vi "reward_behavior_no_TO.vi"() -> ()   [LabVIEW 2019]
doc: "The myRIO Project template acquires acceleration data from the onboard accelerometer and displays the changes of acceleration values in a waveform chart."
uses:
  <vilib>/Analysis/Matrix/Datatypes/RealMatrix.ctl
  <vilib>/myRIO/Common/Instrument Driver Framework/myRIO v1.0/Encoder/typedefs/Encoder Signal Mode.ctl
  <vilib>/myRIO/Instrument Drivers/Onboard IO/Encoder/typedefs/Encoder Reference.ctl
  <vilib>/myRIO/Common/Instrument Driver Framework/Utilities/typedefs/myRIO Generic Hardware Reference.ctl
  <vilib>/myRIO/Common/Instrument Driver Framework/Utilities/typedefs/Hardware Version Enum.ctl
  <vilib>/myRIO/Common/Instrument Driver Framework/Utilities/typedefs/myRIO v1.0 Reference.ctl
  <vilib>/myRIO/Common/Instrument Driver Framework/Utilities/typedefs/Generic FPGA Reference.ctl
  <vilib>/myRIO/Common/Instrument Driver Framework/myRIO v1.0/Encoder/typedefs/Encoder Channels Enum.ctl
  <vilib>/myRIO/Common/Instrument Driver Framework/myRIO v1.0/Encoder/typedefs/Encoder Configuration v1.0.ctl
  <vilib>/userdefined/High Color/nirio_resource_hc.ctl
  <vilib>/myRIO/Instrument Drivers/Onboard IO/DIO/typedefs/DIO Reference.ctl
  <vilib>/myRIO/Common/Instrument Driver Framework/myRIO v1.0/DIO/typedefs/DIO Channels List.ctl
  <vilib>/myRIO/Common/Instrument Driver Framework/myRIO v1.0/DIO/typedefs/DIO Channels Enum.ctl
  <vilib>/myRIO/Common/Instrument Driver Framework/Utilities/vis/Is FPGA Ref Available.vi
  <vilib>/myRIO/Common/Instrument Driver Framework/myRIO v1.0/Encoder/vis/myRIO v1.1 Open Encoder.vi
  <vilib>/myRIO/Instrument Drivers/Onboard IO/Encoder/vis/Read.vi
  <vilib>/myRIO/Common/Instrument Driver Framework/myRIO v1.0/DIO/vis/myRIO v1.1 Open DIO.vi
  <vilib>/myRIO/Instrument Drivers/Onboard IO/DIO/vis/Write.vi
  <vilib>/myRIO/Instrument Drivers/Onboard IO/DIO/vis/Read.vi
  <vilib>/myRIO/Common/Instrument Driver Framework/Utilities/vis/Validate Channels.vi
  <vilib>/myRIO/Common/Instrument Driver Framework/myRIO v1.0/Encoder/vis/myRIO v1.0 Reserve Encoder.vi
  <vilib>/myRIO/Common/Instrument Driver Framework/myRIO v1.0/DIO/vis/myRIO v1.0 Reserve DIO.vi
  <vilib>/myRIO/Common/Instrument Driver Framework/myRIO v1.0/Encoder/vis/myRIO v1.0 Build MUX Configuration Encoder.vi
  <vilib>/myRIO/Common/Instrument Driver Framework/myRIO v1.0/Resource Manager/vis/myRIO v1.0 Reserve Channel List.vi
  <vilib>/myRIO/Common/Instrument Driver Framework/myRIO v1.0/DIO/vis/myRIO v1.0 Build MUX Configuration DIO.vi
  <vilib>/myRIO/Common/Instrument Driver Framework/myRIO v1.0/Resource Manager/vis/myRIO v1.0 Create Configuration List.vi
  <vilib>/myRIO/Common/Instrument Driver Framework/myRIO v1.0/Resource Manager/vis/myRIO v1.0 Reserve Channel.vi
  <vilib>/myRIO/Common/Instrument Driver Framework/myRIO v1.0/Resource Manager/vis/myRIO v1.0 Unreserve Channel.vi
  <vilib>/myRIO/Common/Instrument Driver Framework/myRIO v1.0/Resource Manager/vis/myRIO v1.0 Build Mutex Name.vi
  <vilib>/Utility/VariantDataType/GetNumericInfo.vi
  <vilib>/Utility/error.llb/Error Cluster From Error Code.vi
  <vilib>/myRIO/Common/Instrument Driver Framework/myRIO v1.0/myRIO v1.1 Open.vi
  <vilib>/myRIO/Common/Instrument Driver Framework/Utilities/vis/IO Manager.vi
  <vilib>/myRIO/Common/Instrument Driver Framework/Utilities/vis/Configuration Manager.vi
  <vilib>/myRIO/Common/Instrument Driver Framework/myRIO v1.0/Resource Manager/vis/myRIO v1.0 Configure IO.vi
  <vilib>/myRIO/Common/Instrument Driver Framework/myRIO v1.0/myRIO v1.0 Close.vi
  <vilib>/myRIO/Common/Instrument Driver Framework/myRIO v1.0/Encoder/vis/myRIO v1.0 Configure Encoder.vi
  <vilib>/myRIO/Common/Instrument Driver Framework/myRIO v1.0/Encoder/vis/myRIO v1.0 Read Encoder.vi
  <vilib>/myRIO/Common/Instrument Driver Framework/myRIO v1.0/DIO/vis/myRIO v1.0 Read DIO.vi
  <vilib>/myRIO/Common/Instrument Driver Framework/myRIO v1.0/DIO/vis/myRIO v1.0 Write DIO.vi
  <vilib>/myRIO/Express VI/Onboard IO/Encoder/Encoder Express VI.xnode
  <vilib>/myRIO/Instrument Drivers/Onboard IO/Encoder/vis/myRIO Encoder Open.xnode
  <vilib>/myRIO/Express VI/Onboard IO/DI/DI Express VI.xnode
  <vilib>/myRIO/Instrument Drivers/Onboard IO/DIO/vis/myRIO DIO Open.xnode
  <vilib>/myRIO/Express VI/Onboard IO/DO/DO Express VI.xnode
  <vilib>/myRIO/Instrument Drivers/Onboard IO/Encoder/Encoder.lvlib
  <vilib>/myRIO/Instrument Drivers/Onboard IO/DIO/DIO.lvlib
  <vilib>/Analysis/Matrix/NI_Matrix.lvlib
panel:
  out "Timings":dbl[](array[numeric])
  out "ISI":dbl
  out "ISI start time":dbl
  out "Time_out":bool=TRUE
  out "Time since lick":dbl
  out "Time of last lick":dbl
  out "Rewarded trials":dbl[](array[numeric])
  out "Rewards":u16
  out "Active Trial":bool
  out "Array temp2":T1
  out "Stimuli Loaded":bool
  out "Stim_ID":dbl[](array[numeric])
  out "Reward_mat":dbl[](array[numeric])
  out "Reward":bool=TRUE
  out "Frame clock":i32
  out "Licks":u32
  out "Lick":bool
  out "Time":dbl
  out "Stop":bool
  in  "Frames to collect":u32
  out "Overflow?":bool
  out "Counter Value":i32
  out "Velocity":dbl
  out "Velocity Plot":dbl[](graph)
  out "Velocity array":dbl[](array[numeric])
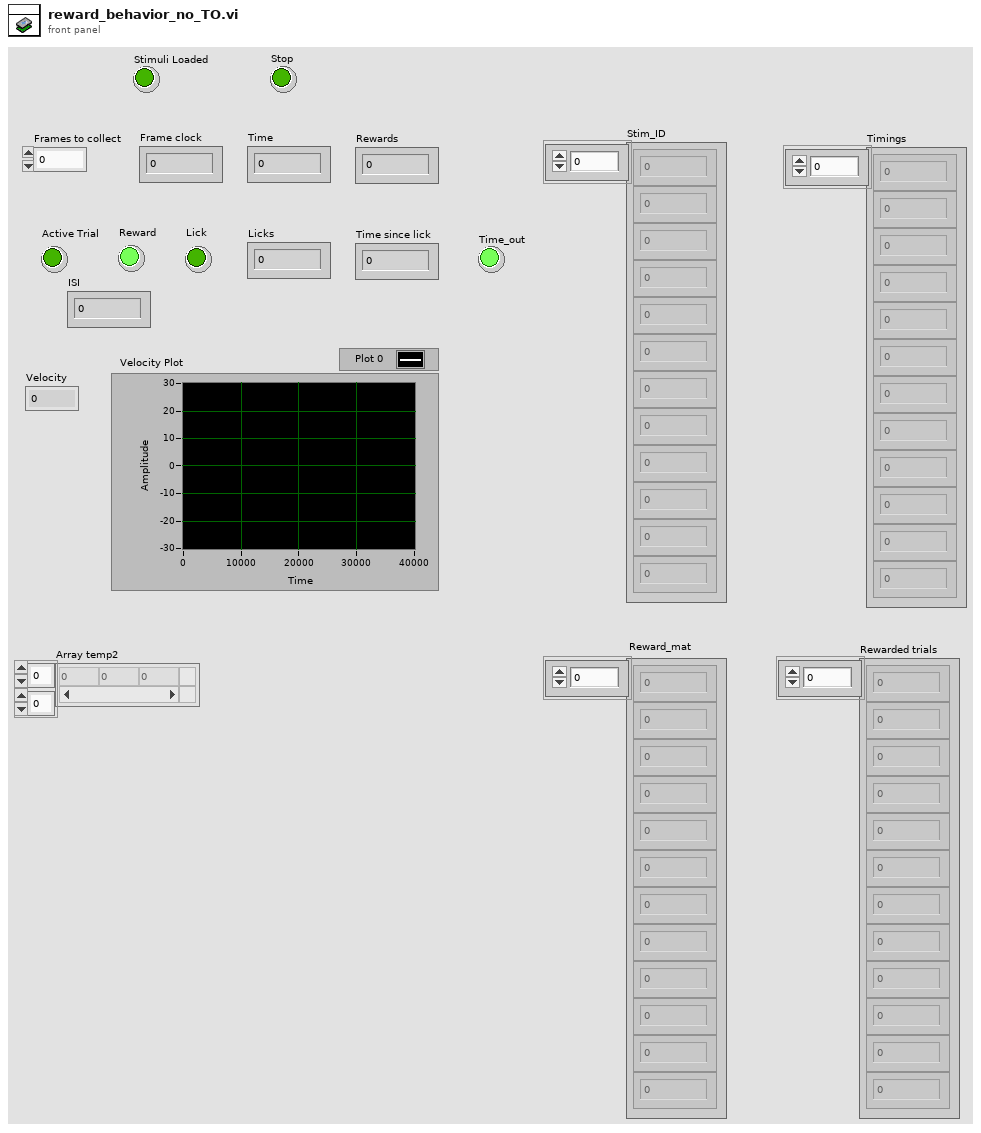
[diagram p1: front panel]
types:
  T1 = typedef "NI_Matrix.lvlib/RealMatrix.ctl" = dbl[][]
  T2 = typedef "Encoder.lvlib/Encoder Reference.ctl" = cluster{"myRIO Reference":T3, "Encoder Channels Enum":T7}
  T3 = typedef "myRIO Generic Hardware Reference.ctl" = cluster{"myRIO Model":T4, "myRIO Hardware Reference":T5}
  T4 = typedef "Hardware Version Enum.ctl" = enum16{"Unknown", "myRIO-1900", "myRIO-1950", "roboRIO", "NI ELVIS RIO CM", "ELVIS III"}
  T5 = typedef "myRIO v1.0 Reference.ctl" = cluster{"Generic FPGA Reference":T6, "Allow multiple opens":bool}
  T6 = typedef "Generic FPGA Reference.ctl" = refnum<k20>
  T7 = typedef "Encoder Channels Enum.ctl" = enum16{"Not Connected", "C/ENC0", "C/ENC1", "A/ENC", "A/ENC0", "A/ENC1", "A/ENC2", "A/ENC3", "A/ENC4", "A/ENC5", "A/ENC6", "A/ENC7", "A/ENC8", "A/ENC9", "B/ENC", "B/ENC0", "B/ENC1", "B/ENC2", "B/ENC3", "B/ENC4", "B/ENC5", "B/ENC6", "B/ENC7", "B/ENC8", "B/ENC9", "DIO/ENC0", "DIO/ENC1", "DIO/ENC2", "DIO/ENC3", "DIO/ENC4"}
  T8 = typedef "Encoder Signal Mode.ctl" = enum16{"Quadrature phase signal", "Step and direction signal"}
  T9 = typedef "nirio_resource_hc.ctl" = tag
  T10 = typedef "DIO.lvlib/DIO Reference.ctl" = cluster{"myRIO Reference":T3, "DIO Channels List":T11}
  T11 = typedef "DIO Channels List.ctl" = T12[]
  T12 = typedef "DIO Channels Enum.ctl" = enum16{"Not Connected", "C/DIO0", "C/DIO1", "C/DIO2", "C/DIO3", "C/DIO4", "C/DIO5", "C/DIO6", "C/DIO7", "A/DIO0", "A/DIO1", "A/DIO2", "A/DIO3", "A/DIO4", "A/DIO5", "A/DIO6", "A/DIO7", "A/DIO8", "A/DIO9", "A/DIO10", "A/DIO11", "A/DIO12", "A/DIO13", "A/DIO14", "A/DIO15", "A/DIO16", "A/DIO17", "A/DIO18", "A/DIO19", "B/DIO0", "B/DIO1", "B/DIO2", "B/DIO3", "B/DIO4", "B/DIO5", "B/DIO6", "B/DIO7", "B/DIO8", "B/DIO9", "B/DIO10", "B/DIO11", "B/DIO12", "B/DIO13", "B/DIO14", "B/DIO15", "B/DIO16", "B/DIO17", "B/DIO18", "B/DIO19", "LED0", "LED1", "LED2", "LED3", "Button0", "DIO/DIO0", "DIO/DIO1", "DIO/DIO2", "DIO/DIO3", "DIO/DIO4", "DIO/DIO5", "DIO/DIO6", "DIO/DIO7", "DIO/DIO8", "DIO/DIO9", "SPI/CS0", "SPI/CS1", "SPI/CS2", "SPI/CS3", "LED RADIO (Green)", "LED RADIO (Red)", "LED COMM (Green)", "LED COMM (Red)", "LED MODE (Green)", "LED MODE (Red)"}
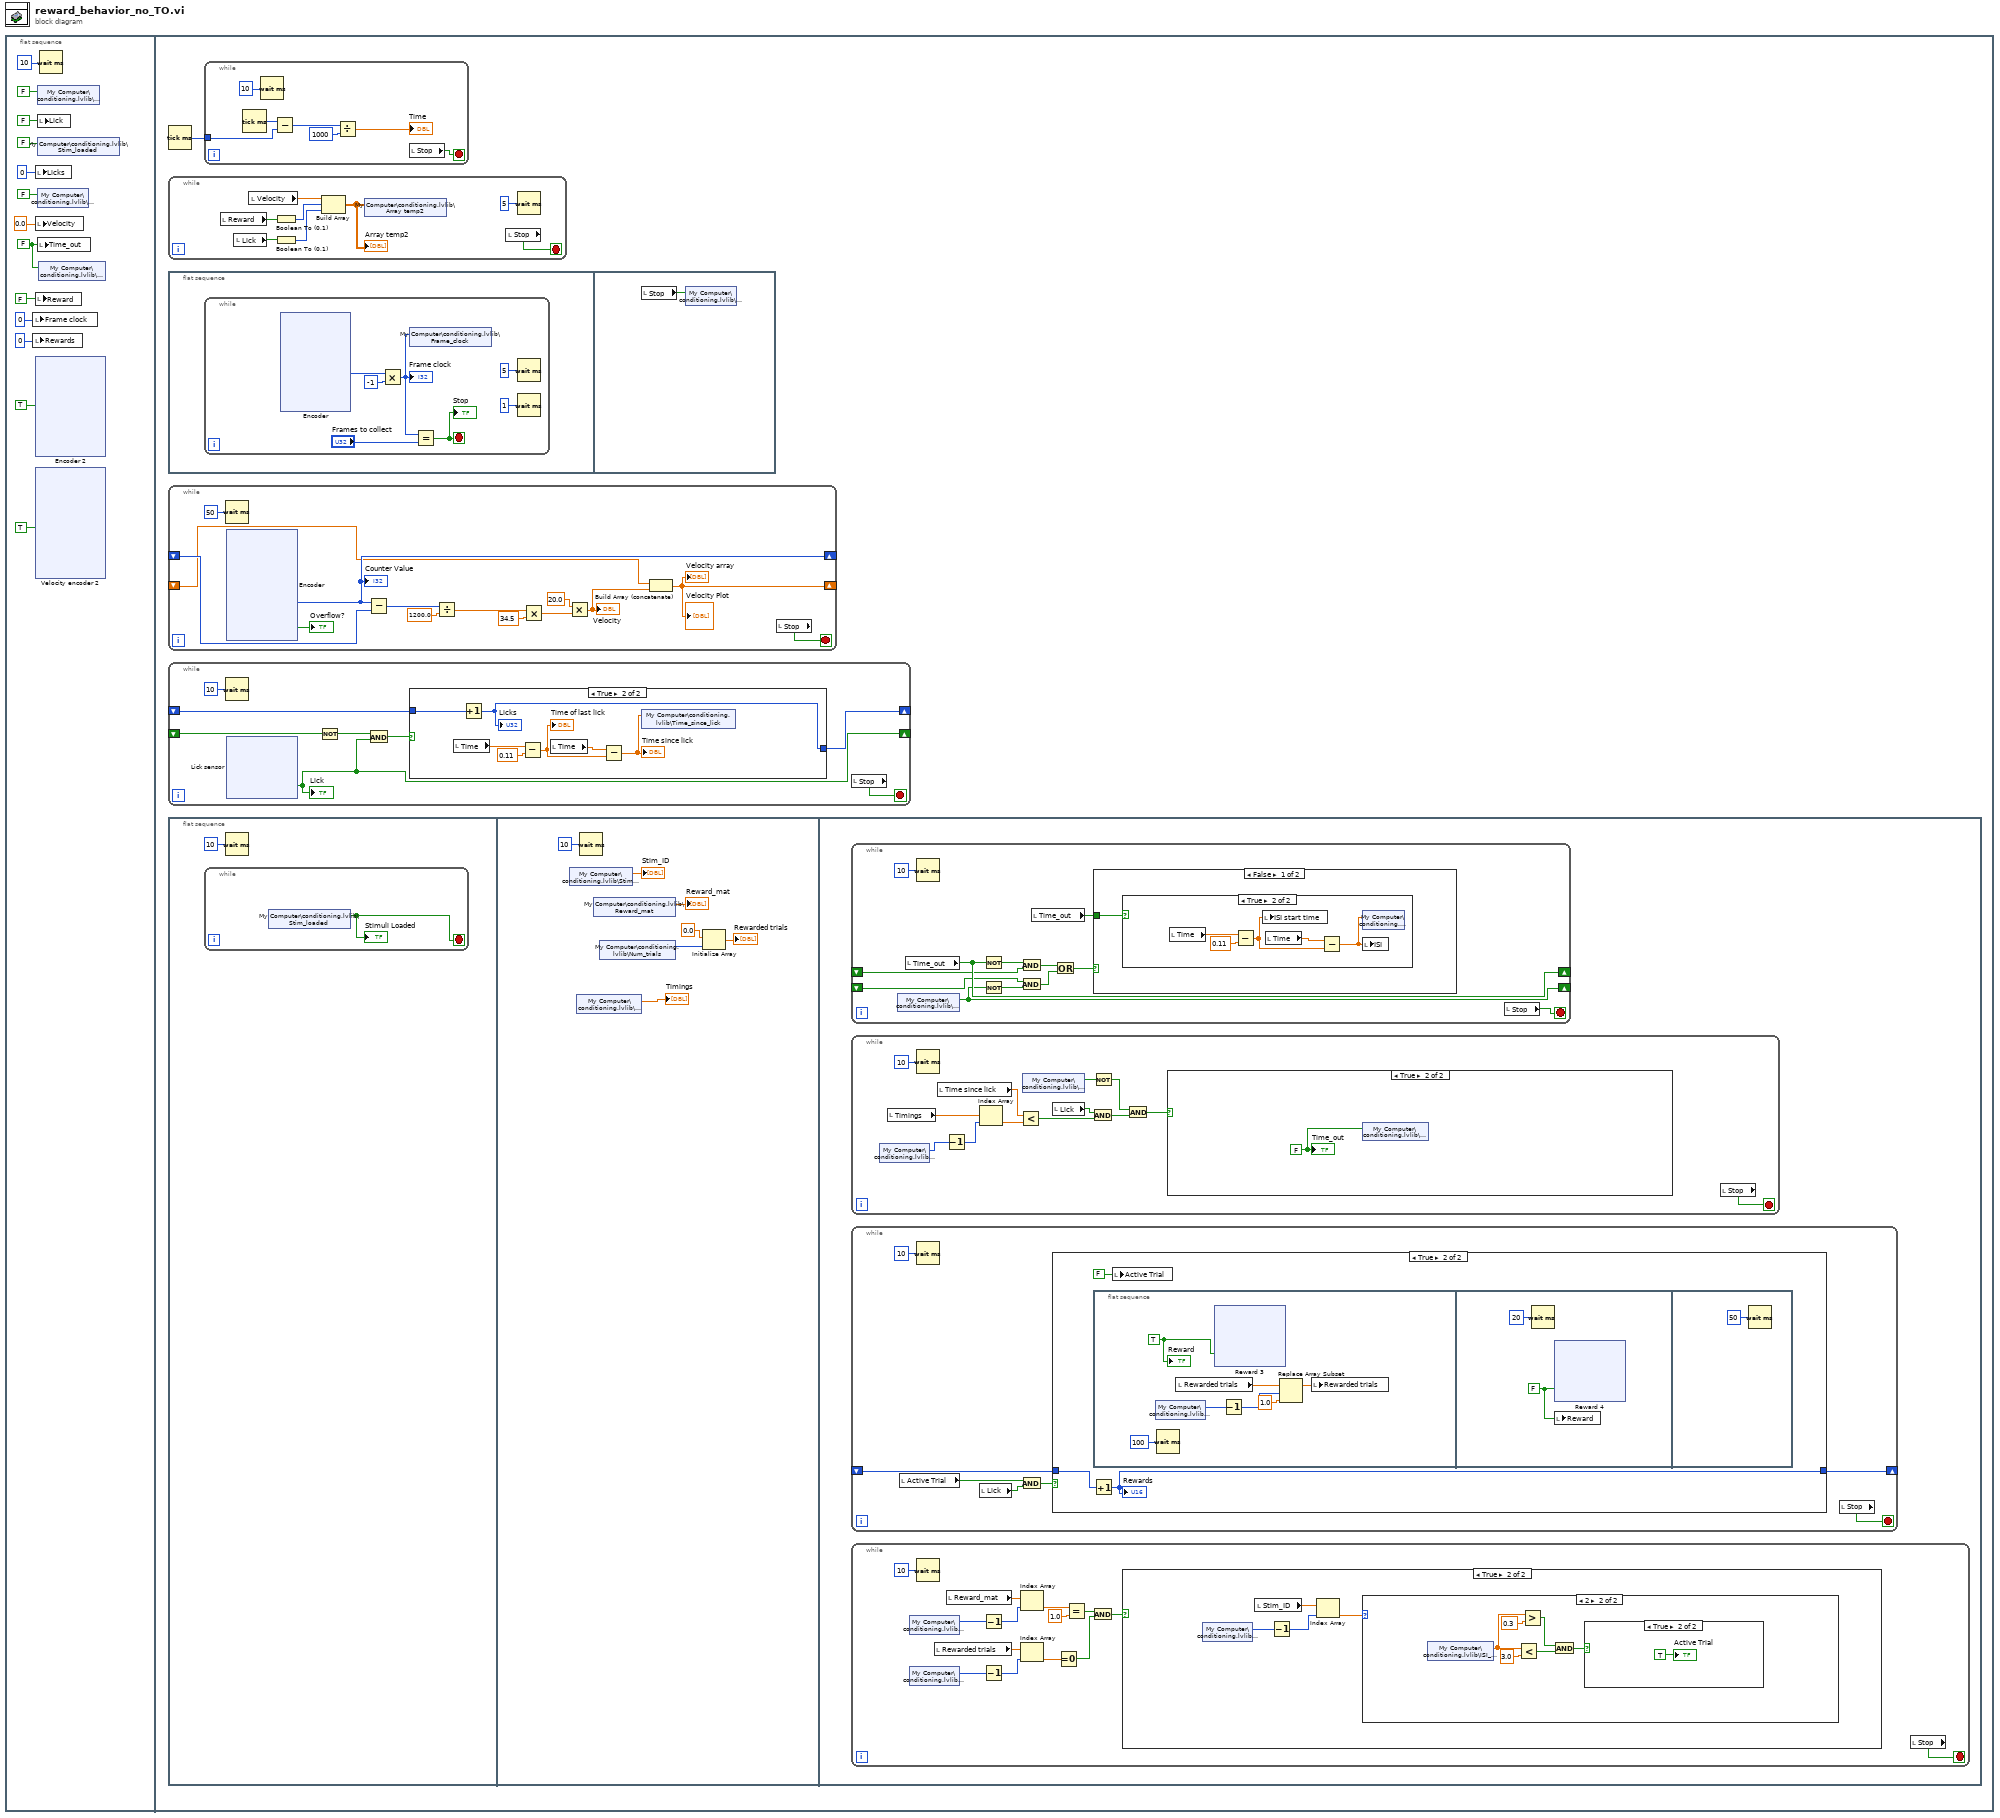
[diagram p0: block diagram]
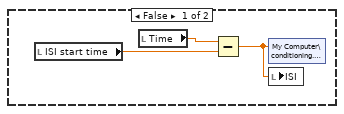
[diagram p3: hidden frame]
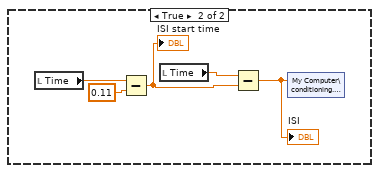
[diagram p4: hidden frame]
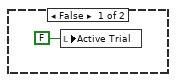
[diagram p5: hidden frame]
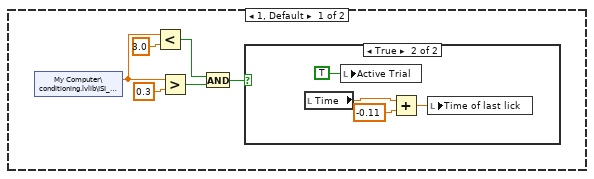
[diagram p6: hidden frame]
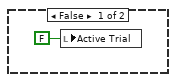
[diagram p7: hidden frame]
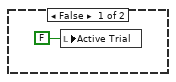
[diagram p8: hidden frame]
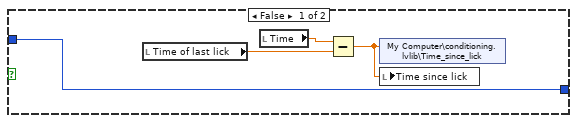
[diagram p10: hidden frame]
diagram:
  n1 = flat-sequence {
    frame #0 {
      w1 = FALSE ("Time_out")
      n2 = local write "Frame clock"(u32 0 ("Frames")) -> ()
      n3 = local write "Rewards"(u16 0 ("Rewards")) -> ()
      n4 = local write "Licks"(u32 0 ("Licks")) -> ()
      n5 = local write "Velocity"(0.0 ("Velocity")) -> ()
      n6 = local write "Reward"(FALSE ("Give reward")) -> ()
      n7 = xnode "Encoder 2"("Reset Counter"=TRUE) -> ()  [unwired: 1 in, 4 out]
      n8 = xnode "Velocity encoder 2"("Reset Counter"=TRUE) -> ()  [unwired: 1 in, 4 out]
      n9 = shared-variable "My Computer\\conditioning.lvlib\\Display"(FALSE ("Display")) -> ()  [unwired: 1 in, 1 out]
      n10 = local write "Lick"(FALSE ("Lick")) -> ()
      n11 = shared-variable "My Computer\\conditioning.lvlib\\Stim_loaded"(FALSE ("Stim_loaded")) -> ()  [unwired: 1 in, 1 out]
      n12 = shared-variable "My Computer\\conditioning.lvlib\\Stop"(FALSE ("Stop")) -> ()  [unwired: 1 in, 1 out]
      n13 = local write "Time_out"(w1) -> ()
      n14 = shared-variable "My Computer\\conditioning.lvlib\\Timeout"(w1) -> ()  [unwired: 1 in, 1 out]
      n15 = Wait (ms)(milliseconds to wait=u32 10) -> ()  [unwired: 1 out]
    }
    frame #1 {
      n16 = Tick Count (ms)() -> (millisecond timer value=w106:u32)
      n17 = while {
        stop <- w108 stop-if-true
        n18 = local read "Reward"() -> (w113:bool)
        n19 = local read "Lick"() -> (w114:bool)
        n20 = local read "Velocity"() -> (w112:dbl)
        n21 = Boolean To (0,1)(Boolean=w113) -> (0, 1=w111:i16)
        n22 = Boolean To (0,1)(Boolean=w114) -> (0, 1=w110:i16)
        n23 = Build Array(w112, w111, w110) -> (w107:T1)
        "Array temp2" <- w107
        n24 = shared-variable "My Computer\\conditioning.lvlib\\Array temp2"(w107) -> ()  [unwired: 1 in, 1 out]
        n25 = local read "Stop"() -> (w108:bool)
        n26 = Wait (ms)(milliseconds to wait=u32 5) -> ()  [unwired: 1 out]
      }
      n27 = flat-sequence {
        frame #0 {
          n28 = while {
            stop <- w294 stop-if-true
            n29 = xnode "Encoder"() -> ("Counter Value"=w298:i32)  [unwired: 2 in, 3 out]
            n30 = Multiply(x=w298, y=-1) -> (x*y=w293:i32)
            "Frame clock" <- w293
            n31 = shared-variable "My Computer\\conditioning.lvlib\\Frame_clock"(w293) -> ()  [unwired: 1 in, 1 out]
            n32 = Equal?(x=w293, y="Frames to collect") -> (x = y?=w294:bool)
            "Stop" <- w294
            n33 = Wait (ms)(milliseconds to wait=u32 5) -> ()  [unwired: 1 out]
            n34 = Wait (ms)(milliseconds to wait=u32 1) -> ()  [unwired: 1 out]
          }
        }
        frame #1 {
          n35 = local read "Stop"() -> (w346:bool)
          n36 = shared-variable "My Computer\\conditioning.lvlib\\Stop"(w346) -> ()  [unwired: 1 in, 1 out]
        }
      }
      n37 = while {
        shift-right: [w411] -> _
        shift-left: _ -> [w412]
        shift-right: [w403] -> _
        shift-left: _ -> [w402]
        stop <- w401 stop-if-true
        n38 = Wait (ms)(milliseconds to wait=u32 50) -> ()  [unwired: 1 out]
        n39 = xnode "Encoder"() -> ("Counter Value"=w411:i32, "Overflow?"=→"Overflow?":bool)  [unwired: 2 in, 2 out]
        "Counter Value" <- w411
        n40 = Subtract(x=w411, y=w412) -> (x-y=w404:i32)
        n41 = Divide(x=w404, y=1200.0 ("600")) -> (x/y=w409:dbl)
        n42 = Multiply(x=w409, y=34.5) -> (x*y=w407:dbl)
        n43 = Multiply(x=20.0, y=w407) -> (x*y=w405:dbl)
        "Velocity" <- w405
        n44 = Build Array (concatenate)(w402, w405) -> (w403:dbl[])
        "Velocity Plot" <- w403
        "Velocity array" <- w403
        n45 = local read "Stop"() -> (w401:bool)
      }
      n46 = while {
        shift-right: [w353] -> _
        shift-left: _ -> [w352]
        shift-right: [w347] -> _
        shift-left: _ -> [w350]
        stop <- w351 stop-if-true
        n47 = Wait (ms)(milliseconds to wait=u32 10) -> ()  [unwired: 1 out]
        n48 = xnode "Lick sensor"() -> ("C/DIO1 (DIO1)"=w347:bool)  [unwired: 1 in, 1 out]
        "Lick" <- w347
        n49 = Not(x=w350) -> (.not. x?=w349:bool)
        n50 = And(x=w349, y=w347) -> (x .and. y?=w348:bool)
        n51 = case shown="True" w348 {
          tunnel: [w358 w365] -> w353
          tunnel: w352 -> [w358 w364]
          frame False {
            n52 = local read "Time of last lick"() -> (w356:dbl)
            n53 = local read "Time"() -> (w357:dbl)
            n54 = Subtract(x=w357, y=w356) -> (x-y=w355:dbl)
            n55 = shared-variable "My Computer\\conditioning.lvlib\\Time_since_lick"(w355) -> ()  [unwired: 1 in, 1 out]
            n56 = local write "Time since lick"(w355) -> ()
          }
          frame True {
            n57 = local read "Time"() -> (w361:dbl)
            n58 = Increment(x=w364) -> (x+1=w365:u32)
            "Licks" <- w365
            n59 = Subtract(x=w361, y=0.11) -> (x-y=w359:dbl)
            "Time of last lick" <- w359
            n60 = local read "Time"() -> (w363:dbl)
            n61 = Subtract(x=w363, y=w359) -> (x-y=w362:dbl)
            "Time since lick" <- w362
            n62 = shared-variable "My Computer\\conditioning.lvlib\\Time_since_lick"(w362) -> ()  [unwired: 1 in, 1 out]
          }
        }
        n63 = local read "Stop"() -> (w351:bool)
      }
      n64 = flat-sequence {
        frame #0 {
          n65 = while {
            stop <- w116 stop-if-true
            n66 = shared-variable "My Computer\\conditioning.lvlib\\Stim_loaded"() -> (w116:bool)  [unwired: 1 in, 1 out]
            "Stimuli Loaded" <- w116
          }
          n67 = Wait (ms)(milliseconds to wait=u32 10) -> ()  [unwired: 1 out]
        }
        frame #1 {
          n68 = shared-variable "My Computer\\conditioning.lvlib\\Stim_ID"() -> (→"Stim_ID":dbl[])  [unwired: 1 in, 1 out]
          n69 = shared-variable "My Computer\\conditioning.lvlib\\Timings"() -> (→"Timings":dbl[])  [unwired: 1 in, 1 out]
          n70 = Wait (ms)(milliseconds to wait=u32 10) -> ()  [unwired: 1 out]
          n71 = shared-variable "My Computer\\conditioning.lvlib\\Reward_mat"() -> (→"Reward_mat":dbl[])  [unwired: 1 in, 1 out]
          n72 = shared-variable "My Computer\\conditioning.lvlib\\Num_trials"() -> (w120:u32)  [unwired: 1 in, 1 out]
          n73 = Initialize Array(0.0 ("element"), w120) -> (→"Rewarded trials":dbl[])
        }
        frame #2 {
          n74 = while {
            shift-right: [w148] -> _
            shift-left: _ -> [w146]
            shift-right: [w144] -> _
            shift-left: _ -> [w143]
            stop <- w149 stop-if-true
            n75 = shared-variable "My Computer\\conditioning.lvlib\\Display"() -> (w144:bool)  [unwired: 1 in, 1 out]
            n76 = local read "Time_out"() -> (w148:bool)
            n77 = Wait (ms)(milliseconds to wait=u32 10) -> ()  [unwired: 1 out]
            n78 = Not(x=w148) -> (.not. x?=w147:bool)
            n79 = Not(x=w144) -> (.not. x?=w142:bool)
            n80 = And(x=w147, y=w146) -> (x .and. y?=w141:bool)
            n81 = And(x=w143, y=w142) -> (x .and. y?=w140:bool)
            n82 = local read "Time_out"() -> (w145:bool)
            n83 = Or(x=w141, y=w140) -> (x .or. y?=w139:bool)
            n84 = case shown="False" w139 {
              tunnel: w145 -> [w150 _]
              frame False {
                n85 = case shown="True" w150 {
                  frame False {
                    n86 = local read "ISI start time"() -> (w153:dbl)
                    n87 = local read "Time"() -> (w152:dbl)
                    n88 = Subtract(x=w152, y=w153) -> (x-y=w151:dbl)
                    n89 = shared-variable "My Computer\\conditioning.lvlib\\ISI"(w151) -> ()  [unwired: 1 in, 1 out]
                    n90 = local write "ISI"(w151) -> ()
                  }
                  frame True {
                    n91 = local read "Time"() -> (w158:dbl)
                    n92 = Subtract(x=w158, y=0.11) -> (x-y=w155:dbl)
                    n93 = local write "ISI start time"(w155) -> ()
                    n94 = local read "Time"() -> (w156:dbl)
                    n95 = Subtract(x=w156, y=w155) -> (x-y=w154:dbl)
                    n96 = shared-variable "My Computer\\conditioning.lvlib\\ISI"(w154) -> ()  [unwired: 1 in, 1 out]
                    n97 = local write "ISI"(w154) -> ()
                  }
                }
              }
              frame True {
                n98 = local read "Time"() -> (w163:dbl)
                n99 = Subtract(x=w163, y=0.11) -> (x-y=w160:dbl)
                "ISI start time" <- w160
                n100 = local read "Time"() -> (w161:dbl)
                n101 = Subtract(x=w161, y=w160) -> (x-y=w159:dbl)
                "ISI" <- w159
                n102 = shared-variable "My Computer\\conditioning.lvlib\\ISI"(w159) -> ()  [unwired: 1 in, 1 out]
              }
            }
            n103 = local read "Stop"() -> (w149:bool)
          }
          n104 = while {
            stop <- w136 stop-if-true
            n105 = shared-variable "My Computer\\conditioning.lvlib\\Trial"() -> (w125:u32)  [unwired: 1 in, 1 out]
            n106 = local read "Timings"() -> (w127:dbl[])
            n107 = Wait (ms)(milliseconds to wait=u32 10) -> ()  [unwired: 1 out]
            n108 = local read "Time since lick"() -> (w135:dbl)
            n109 = Decrement(x=w125) -> (x-1=w124:u32)
            n110 = Index Array(array=w127, index=w124) -> (element=w126:dbl)
            n111 = Less?(x=w135, y=w126) -> (x < y?=w134:bool)
            n112 = shared-variable "My Computer\\conditioning.lvlib\\Display"() -> (w131:bool)  [unwired: 1 in, 1 out]
            n113 = local read "Lick"() -> (w133:bool)
            n114 = Not(x=w131) -> (.not. x?=w130:bool)
            n115 = And(x=w133, y=w134) -> (x .and. y?=w129:bool)
            n116 = And(x=w130, y=w129) -> (x .and. y?=w128:bool)
            n117 = case shown="True" w128 {
              frame False {
              }
              frame True {
                w137 = FALSE
                n118 = shared-variable "My Computer\\conditioning.lvlib\\Timeout"(w137) -> ()  [unwired: 1 in, 1 out]
                "Time_out" <- w137
              }
            }
            n119 = local read "Stop"() -> (w136:bool)
          }
          n120 = while {
            shift-right: [w205] -> _
            shift-left: _ -> [w204]
            stop <- w208 stop-if-true
            n121 = local read "Active Trial"() -> (w202:bool)
            n122 = Wait (ms)(milliseconds to wait=u32 10) -> ()  [unwired: 1 out]
            n123 = local read "Lick"() -> (w203:bool)
            n124 = And(x=w202, y=w203) -> (x .and. y?=w206:bool)
            n125 = case shown="True" w206 {
              tunnel: [w209 w212] -> w205
              tunnel: w204 -> [w209 w211]
              frame False {
              }
              frame True {
                n126 = Increment(x=w211) -> (x+1=w212:u16)
                "Rewards" <- w212
                n127 = flat-sequence {
                  frame #0 {
                    w218 = TRUE ("C/DIO0 (DIO0)")
                    n128 = shared-variable "My Computer\\conditioning.lvlib\\Trial"() -> (w217:u32)  [unwired: 1 in, 1 out]
                    n129 = Wait (ms)(milliseconds to wait=u32 100) -> ()  [unwired: 1 out]
                    n130 = local read "Rewarded trials"() -> (w215:dbl[])
                    n131 = xnode "Reward 3"("C/DIO0 (DIO0)"=w218) -> ()  [unwired: 1 in, 1 out]
                    n132 = Decrement(x=w217) -> (x-1=w216:u32)
                    n133 = Replace Array Subset(array=w215, new element=1.0 ("new element/subarray"), index=w216) -> (w213:dbl[])
                    n134 = local write "Rewarded trials"(w213) -> ()
                    "Reward" <- w218
                  }
                  frame #1 {
                    w256 = FALSE ("C/DIO0 (DIO0)")
                    n135 = Wait (ms)(milliseconds to wait=u32 20) -> ()  [unwired: 1 out]
                    n136 = xnode "Reward 4"("C/DIO0 (DIO0)"=w256) -> ()  [unwired: 1 in, 1 out]
                    n137 = local write "Reward"(w256) -> ()
                  }
                  frame #2 {
                    n138 = Wait (ms)(milliseconds to wait=u32 50) -> ()  [unwired: 1 out]
                  }
                }
                n139 = local write "Active Trial"(FALSE ("Active Trial")) -> ()
              }
            }
            n140 = local read "Stop"() -> (w208:bool)
          }
          n141 = while {
            stop <- w177 stop-if-true
            n142 = shared-variable "My Computer\\conditioning.lvlib\\Trial"() -> (w173:u32)  [unwired: 1 in, 1 out]
            n143 = shared-variable "My Computer\\conditioning.lvlib\\Trial"() -> (w169:u32)  [unwired: 1 in, 1 out]
            n144 = Wait (ms)(milliseconds to wait=u32 10) -> ()  [unwired: 1 out]
            n145 = local read "Rewarded trials"() -> (w170:dbl[])
            n146 = local read "Reward_mat"() -> (w172:dbl[])
            n147 = Decrement(x=w173) -> (x-1=w174:u32)
            n148 = Decrement(x=w169) -> (x-1=w168:u32)
            n149 = Index Array(array=w172, index=w174) -> (element=w175:dbl)
            n150 = Index Array(array=w170, index=w168) -> (element=w167:dbl)
            n151 = Equal To 0?(x=w167) -> (x = 0?=w166:bool)
            n152 = Equal?(x=w175, y=1.0) -> (x = y?=w165:bool)
            n153 = And(x=w165, y=w166) -> (x .and. y?=w164:bool)
            n154 = case shown="True" w164 {
              frame False {
                n155 = local write "Active Trial"(FALSE ("Active_trial")) -> ()
              }
              frame True {
                n156 = shared-variable "My Computer\\conditioning.lvlib\\Trial"() -> (w180:u32)  [unwired: 1 in, 1 out]
                n157 = local read "Stim_ID"() -> (w182:dbl[])
                n158 = Decrement(x=w180) -> (x-1=w181:u32)
                n159 = Index Array(array=w182, index=w181) -> (element=w179:dbl)
                n160 = case shown="2" w179 {
                  frame 1, Default {
                    n161 = shared-variable "My Computer\\conditioning.lvlib\\ISI_Time"() -> (w187:dbl)  [unwired: 1 in, 1 out]
                    n162 = Less?(x=w187, y=3.0) -> (x < y?=w185:bool)
                    n163 = Greater?(x=w187, y=0.3) -> (0:w184:bool)
                    n164 = And(x=w185, y=w184) -> (x .and. y?=w183:bool)
                    n165 = case shown="True" w183 {
                      frame False {
                        n166 = local write "Active Trial"(FALSE ("Active Trial")) -> ()
                      }
                      frame True {
                        n167 = local read "Time"() -> (w192:dbl)
                        n168 = local write "Active Trial"(TRUE ("Active Trial")) -> ()
                        n169 = Add(x=w192, y=-0.11) -> (x+y=w190:dbl)
                        n170 = local write "Time of last lick"(w190) -> ()
                      }
                    }
                  }
                  frame 2 {
                    n171 = shared-variable "My Computer\\conditioning.lvlib\\ISI_Time"() -> (w198:dbl)  [unwired: 1 in, 1 out]
                    n172 = Less?(x=w198, y=3.0) -> (x < y?=w195:bool)
                    n173 = Greater?(x=w198, y=0.3) -> (0:w196:bool)
                    n174 = And(x=w196, y=w195) -> (x .and. y?=w194:bool)
                    n175 = case shown="True" w194 {
                      frame False {
                        n176 = local write "Active Trial"(FALSE ("Active Trial")) -> ()
                      }
                      frame True {
                        "Active Trial" <- TRUE ("Active Trial")
                      }
                    }
                  }
                }
              }
            }
            n177 = local read "Stop"() -> (w177:bool)
          }
        }
      }
      n178 = while {
        tunnel: w106 -> [w466]
        stop <- w464 stop-if-true
        n179 = Tick Count (ms)() -> (millisecond timer value=w467:u32)
        n180 = Wait (ms)(milliseconds to wait=u32 10) -> ()  [unwired: 1 out]
        n181 = Subtract(x=w467, y=w466) -> (x-y=w463:u32)
        n182 = Divide(x=w463, y=u32 1000) -> (x/y=→"Time":dbl)
        n183 = local read "Stop"() -> (w464:bool)
      }
    }
  }
